vi "TestStand_Control ( Step-Group - Keyword ).vi"(11 "Step_group":string[](array[string])) -> (3 "Array":T1[](array[typedef]))   [LabVIEW 2018, in "TestStand_Control.lvlib"]
uses:
  TestStand_Control.lvlib
  Module_Controls/TestStand ( KWD_Info ).ctl
  Module_Controls/Keyword_Info ( Data Structure ).ctl
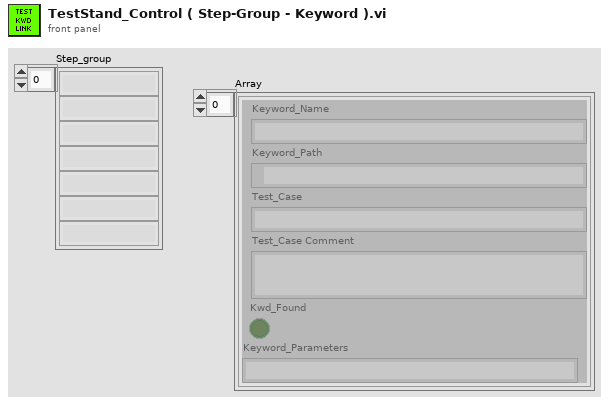
[diagram p1: front panel]
types:
  T1 = typedef "TestStand ( KWD_Info ).ctl" = cluster{"Keyword_Name":string, "Keyword_Path":path, "Test_Case":string, "Test_Case Comment":string, "Kwd_Found":bool, "Keyword_Parameters":string}
  T2 = typedef "Keyword_Info ( Data Structure ).ctl" = cluster{"Name":string, "Path":path, "Keyword_Group":string, "Keyword_Parameters":cluster{"Function":string, "Parameter_List":cluster{"Parameter_Name":string, "Parameter_Type":string, "Parameter_Comment":string, "Required":bool, "Default_Value":string, "Ring_Data":string[]}[]}[]}
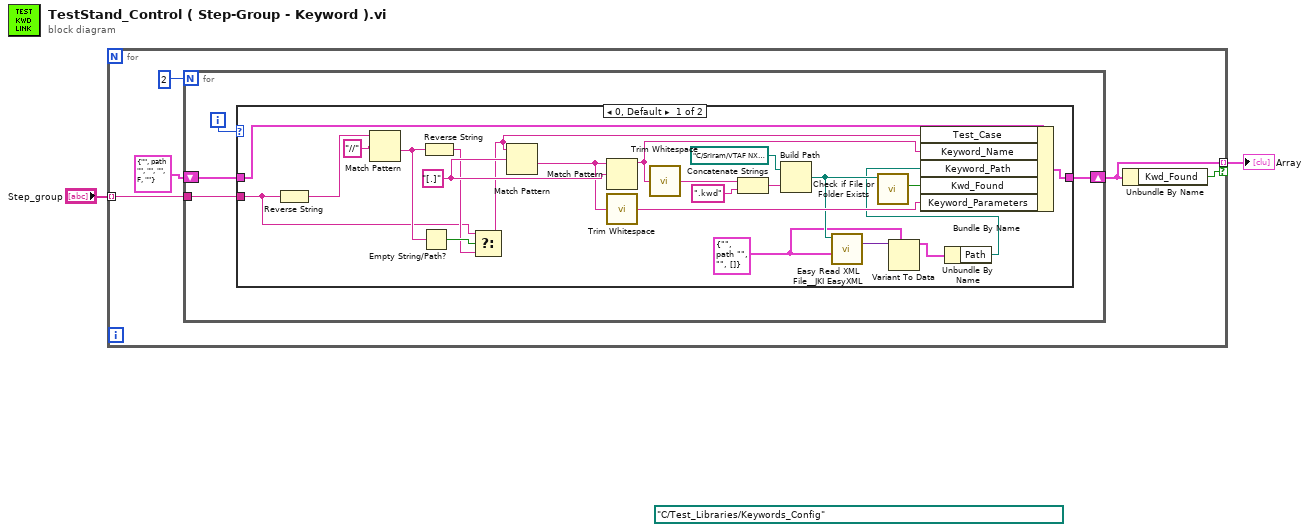
[diagram p0: block diagram]
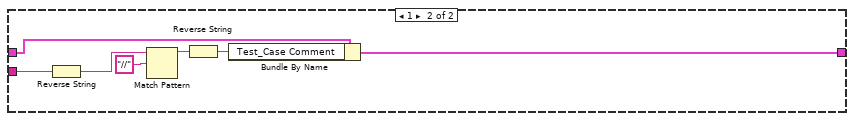
[diagram p2: hidden frame]
diagram:
  (unwired) path "C:/Test_Libraries/Keywords_Config" ("XML File Path")
  n1 = for {
    tunnel: "Step_group" -> [w7] mode=indexing
    tunnel: [w4] -> w2 mode=indexing if=w3
    n2 = for {
      N: 2 -> [_]
      tunnel: w7 -> [w11]
      shift-right: [w8] -> w4
      shift-left: T1 {"Keyword_Name"="", "Keyword_Path"=path "", "Test_Case"="", "Test_Case Comment"="", "Kwd_Found"=FALSE, "Keyword_Parameters"=""} ("Keyword") -> [w9]
      i -> [w10]
      n3 = case shown="0, Default" w10 {
        tunnel: w11 -> [w12 w41]
        tunnel: w9 -> [w34 w38]
        tunnel: [w29 w37] -> w8
        frame 0, Default {
          w19 = T2 {"Name"="", "Path"=path "", "Keyword_Group"="", "Keyword_Parameters"=[]} ("Keyword")
          w33 = "[.]" ("search string")
          n4 = Reverse String(1:w12) -> (0:w26:string)
          n5 = Match Pattern(string=w26, regular expression="//") -> (after substring=w16:string)  [unwired: 1 in, 3 out]
          n6 = Empty String/Path?(string/path=w16) -> (empty?=w15:bool)
          n7 = Reverse String(1:w16) -> (0:w14:string)
          n8 = Select(t=w12, s=w15, f=w14) -> (s? t:f=w13:string)
          n9 = Match Pattern(string=w13, regular expression=w33) -> (after substring=w23:string)  [unwired: 1 in, 3 out]
          n10 = Match Pattern(string=w23, regular expression=w33) -> (before substring=w28:string)  [unwired: 1 in, 3 out]
          n11 = call <vilib>:"Trim Whitespace.vi"("string"=w23) -> ("trimmed string"=w22:string)  [unwired: 1 in]
          n12 = call <vilib>:"Trim Whitespace.vi"("string"=w28) -> ("trimmed string"=w24:string)  [unwired: 1 in]
          n13 = Concatenate Strings(w24, ".kwd" ("string")) -> (w32:string)
          n14 = Build Path(base path=path "C:/Sriram/VTAF NXG/IOT Devices/test-automation/Libraries/Test_Libraries/Keywords_Config" ("XML File Path"), name or relative path=w32) -> (appended path=w21:path)
          n15 = call <vilib>:"Easy Read XML File__JKI EasyXML.vi"("LabVIEW Data (Type)"=w19, "XML File Path"=w21) -> ("LabVIEW Data"=w20:variant)  [unwired: 7 in, 2 out]
          n16 = call <vilib>:"Check if File or Folder Exists.vi"("path"=w21) -> ("file or folder exists?"=w27:bool)  [unwired: 8 in, 2 out]
          n17 = Variant To Data(type=w19, Variant=w20) -> (data=w18:T2)  [unwired: 1 in, 1 out]
          n18 = Unbundle By Name(w18) -> ("Path"=w17:path)
          n19 = Bundle By Name(cluster=w34, "Test_Case"=w13, "Keyword_Name"=w28, "Keyword_Path"=w17, "Kwd_Found"=w27, "Keyword_Parameters"=w22) -> (w29:T1)
        }
        frame 1 {
          n20 = Reverse String(1:w41) -> (0:w40:string)
          n21 = Match Pattern(string=w40, regular expression="//") -> (before substring=w36:string)  [unwired: 1 in, 3 out]
          n22 = Reverse String(1:w36) -> (0:w35:string)
          n23 = Bundle By Name(cluster=w38, "Test_Case Comment"=w35) -> (w37:T1)
        }
      }
    }
    n24 = Unbundle By Name(w4) -> ("Kwd_Found"=w3:bool)
  }
  "Array" <- w2
